vi "Jet_Input.vi"(4 "error in (no error)":errorcluster, 5 "Measured origin x,y":dbl[](array[numeric])=[0.83, 0.79], 6 "Element In":T6, 7 "Outputmode":u16(ring) items=["Get Path", "Make Layout", "Create TRJs"]) -> (0 "error out":errorcluster, 1 "Init Cluster":T8, 2 "TRJs":T5, 3 "Elements out":T7(array[cluster]))   [LabVIEW 2009]
panel:
  out "output cluster":T1
  in  "Tab Control":enum32{"Main", "Expert", "Output"}(tab)=enum."Output"
  out "Tube length":dbl=7.947000000000001
  in  "Ab rate tube":dbl=0.016
  in  "Laser interval tube":dbl=0.01
  in  "Hight to groove(tube center)":dbl=3.0
  in  "Origin to jet outlet (Jet toal)":dbl=10.0
  in  "stop":bool
  in  "Machining geometry (mm)":T2={"a0 radius"=0.35, "a0 depth"=0.5, "b0 radius"=0.1, "b0(depth)"=0.15, "a1 radius"=0.2, "a1 depth"=0.3}
  in  "Length":T3={" l0"=0.5, "l1"=0.35, "l 2"=0.5, "l 3"=0.5}
  out "jet head  length":dbl=1.853
  in  "Gap between  \nl1 and l2":dbl=0.003
  in  "Laser interval jet":dbl=0.008
  in  "Ab rate jet":dbl=0.01
  out "Drawing":picture
  in  "XY Line Arc Trajectory tube":T4={"Velocity (units/s)"=3.0, "Acceleration (unts/s2)"=20.0, "Number of times of execution"=1} {"Acceleration (unts/s2)" format="%.6f"; "Velocity (units/s)" format="%.6f"; "Number of times of execution" format="%.6f"}
  in  "XY Line Arc Trajectory jet":T4={"Velocity (units/s)"=3.0, "Acceleration (unts/s2)"=20.0, "Number of times of execution"=1} {"Acceleration (unts/s2)" format="%.6f"; "Velocity (units/s)" format="%.6f"; "Number of times of execution" format="%.6f"}
  in  "Type":i32=2
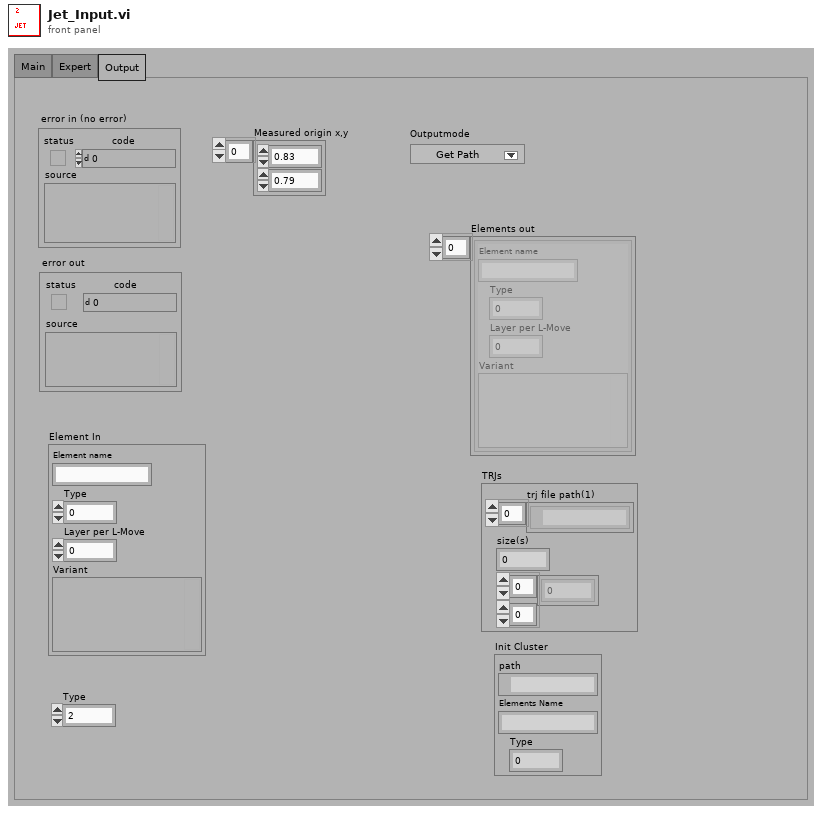
[diagram p1: front panel]
types:
  T1 = cluster{"Hight to groove(tube center)":dbl, "Origin to jet outlet (Jet toal)":dbl, "Laser interval tube":dbl, "Ab rate tube":dbl, "Machining geometry (mm)":cluster{"a0 radius":dbl, "a0 depth":dbl, "b0 radius":dbl, "b0(depth)":dbl, "a1 radius":dbl, "a1 depth":dbl}, "Gap between  \nl1 and l2 ":dbl, "Length":cluster{" l0":dbl, "l1":dbl, "l 2":dbl, "l 3":dbl}, "Laser interval jet":dbl, "Ab rate jet":dbl, "XY Line Arc Trajectory tube":cluster{"Velocity (units/s)":dbl, "Acceleration (unts/s2)":dbl, "Number of times of execution":i32}, "XY Line Arc Trajectory jet":cluster{"Velocity (units/s)":dbl, "Acceleration (unts/s2)":dbl, "Number of times of execution":i32}, "Part #":dbl}
  T2 = cluster{"a0 radius":dbl, "a0 depth":dbl, "b0 radius":dbl, "b0(depth)":dbl, "a1 radius":dbl, "a1 depth":dbl}
  T3 = cluster{" l0":dbl, "l1":dbl, "l 2":dbl, "l 3":dbl}
  T4 = cluster{"Velocity (units/s)":dbl, "Acceleration (unts/s2)":dbl, "Number of times of execution":i32}
  T5 = cluster{"trj file path(1)":path[], "size(s)":i32, dbl[][]}
  T6 = cluster{"Element name":string, "Type":i32, "Layer per L-Move":i32, "Variant":variant}
  T7 = cluster{"Element name":string, "Type":i32, "Layer per L-Move":i32, "Variant":variant}[]
  T8 = cluster{"path":path, "Elements Name":string, "Type":i32}
  T9 = cluster{"path":path, "Button Name":string, "Type":i32}
  T10 = cluster{"Element name":string, "Value":i32, "Layer per L-Move":i32, "Variant":variant}
  T11 = cluster{"Element name":string, "Value":i32, "Layer per L-Move":i32, "Variant":variant}[]
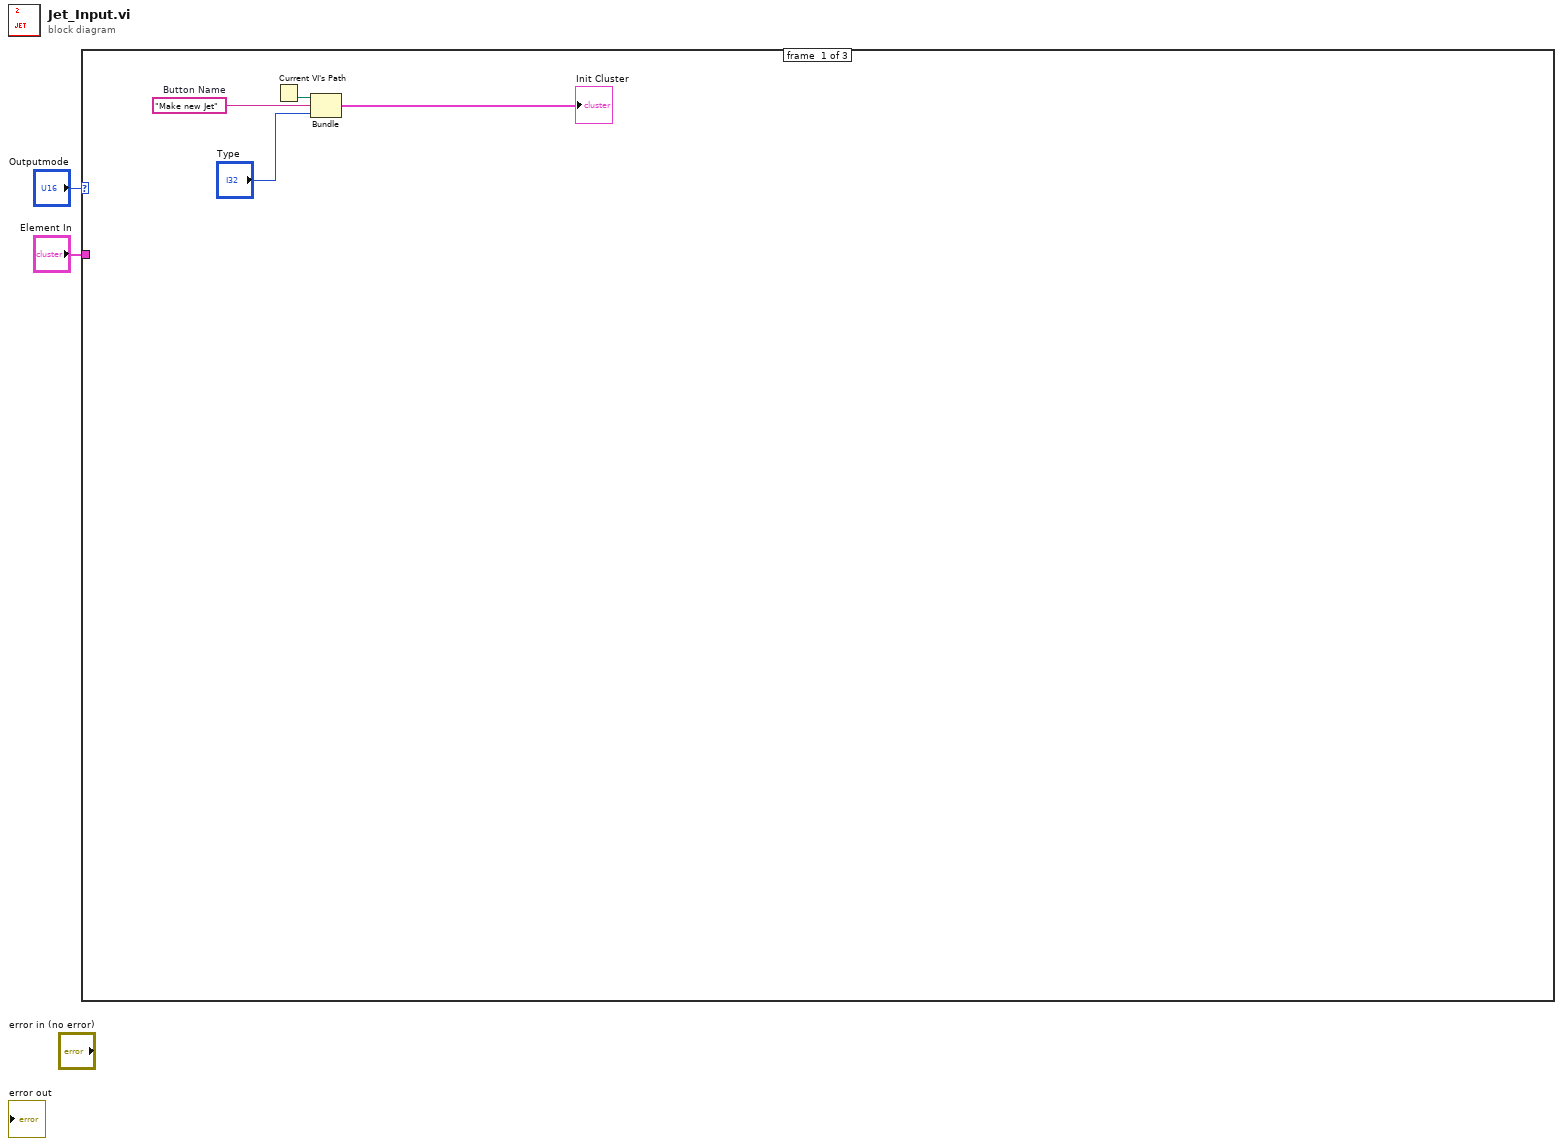
[diagram p0: block diagram]
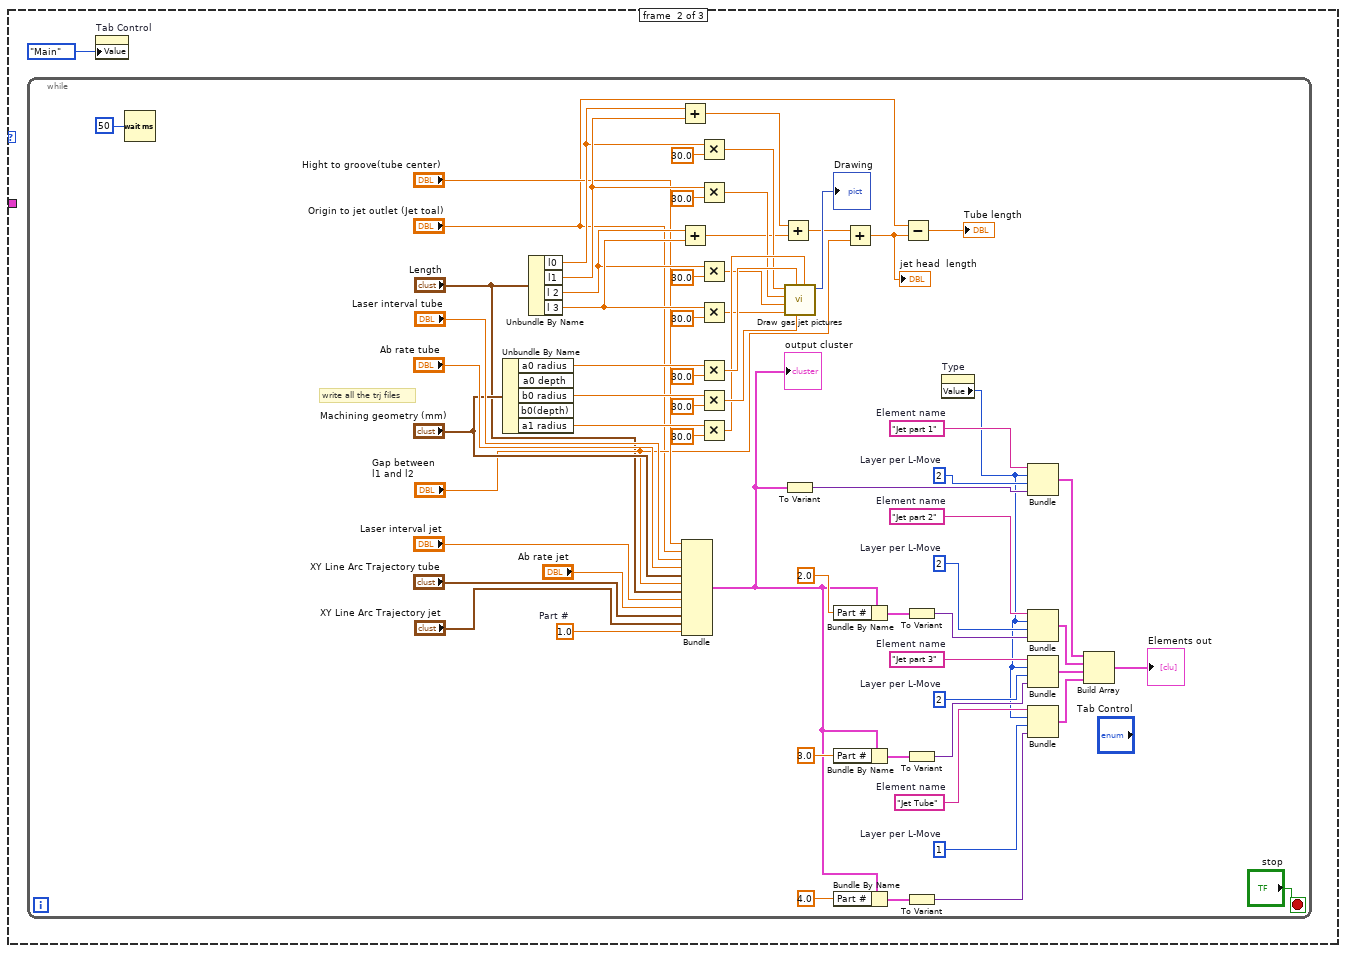
[diagram p2: hidden frame]
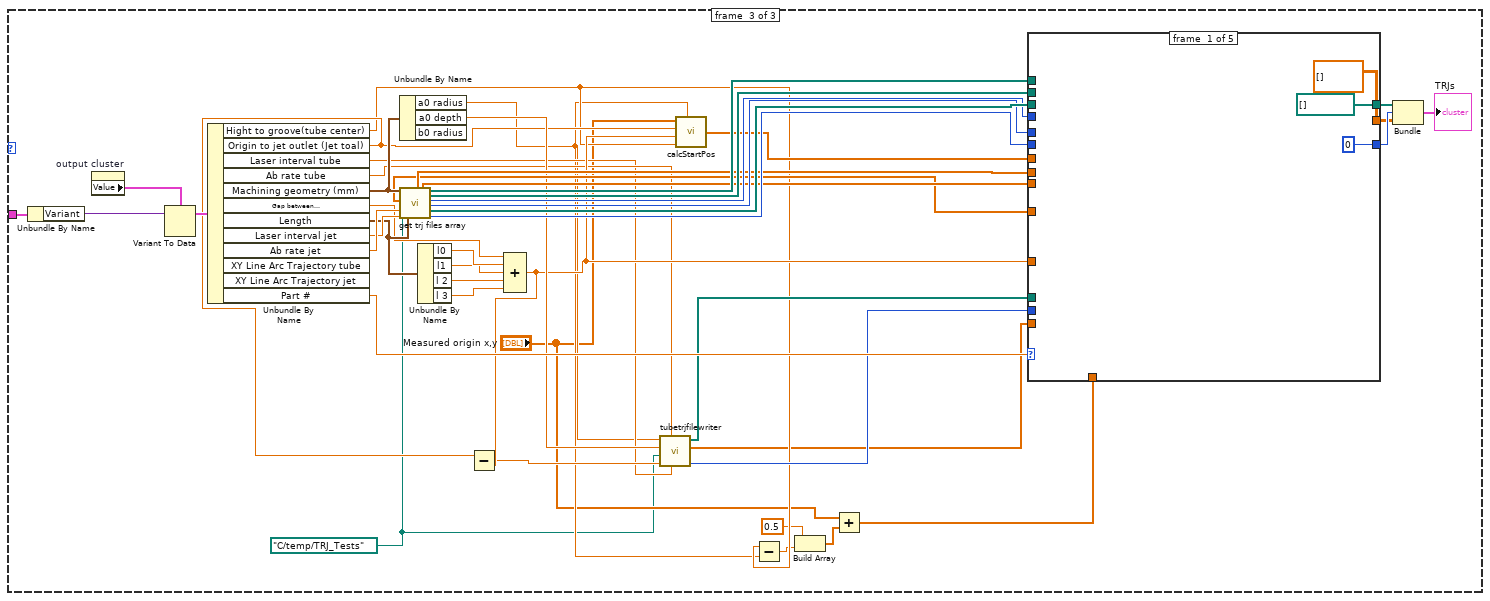
[diagram p3: hidden frame]
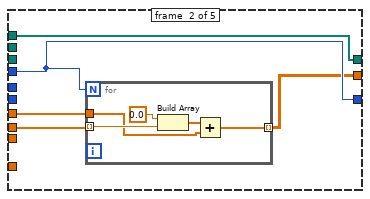
[diagram p4: hidden frame]
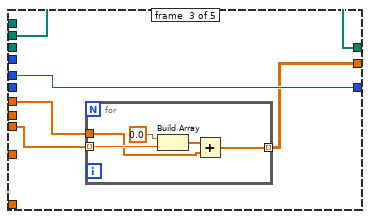
[diagram p5: hidden frame]
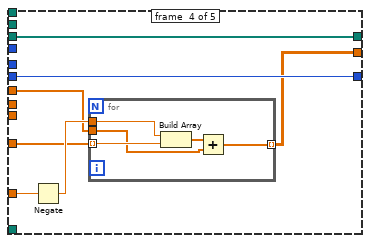
[diagram p6: hidden frame]
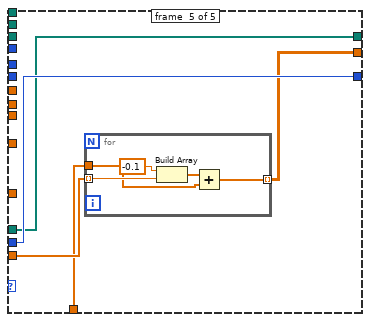
[diagram p7: hidden frame]
diagram:
  n1 = case shown="2" "Outputmode" {
    tunnel: "Element In" -> [_ _ w118]
    frame #0 {
      w6 = "Make new Jet"  # Button Name
      n2 = Current VI's Path() -> (path=w5:path)
      n3 = Bundle("path"=w5, "Button Name"=w6, "Type"="Type") -> (→"Init Cluster":T9)  [unwired: 1 in]
    }
    frame #1 {
      n4 = while {
        stop <- "stop" stop-if-true
        w21 = 1  # Layer per L-Move
        w20 = "Jet Tube"  # Element name
        w22 = 2  # Layer per L-Move
        w23 = "Jet part 3"  # Element name
        w27 = 2  # Layer per L-Move
        w26 = "Jet part 2"  # Element name
        w30 = 1.0  # Part #
        w31 = 2  # Layer per L-Move
        w32 = "Jet part 1"  # Element name
        # "write all the trj files"
        n5 = Wait (ms)(milliseconds to wait=u32 50) -> ()  [unwired: 1 out]
        n6 = Unbundle By Name("Machining geometry (mm)") -> ("a0 radius"=w71:dbl, "b0 radius"=w70:dbl, "a1 radius"=w69:dbl)  [unwired: 2 out]
        n7 = Unbundle By Name("Length") -> ("l0"=w57:dbl, "l1"=w58:dbl, "l 2"=w59:dbl, "l 3"=w60:dbl)
        n8 = Add(x=w57, y=w58) -> (x+y=w47:dbl)
        n9 = Add(x=w59, y=w60) -> (x+y=w48:dbl)
        n10 = Bundle("Hight to groove(tube center)"="Hight to groove(tube center)", "Origin to jet outlet (Jet toal)"="Origin to jet outlet (Jet toal)", "Laser interval tube"="Laser interval tube", "Ab rate tube"="Ab rate tube", "Machining geometry (mm)"="Machining geometry (mm)", "Gap between  \nl1 and l2"="Gap between  \nl1 and l2", "Length"="Length", "Laser interval jet"="Laser interval jet", "Ab rate jet"="Ab rate jet", "XY Line Arc Trajectory tube"="XY Line Arc Trajectory tube", "XY Line Arc Trajectory jet"="XY Line Arc Trajectory jet", "Part #"=w30) -> (w13:T1)  [unwired: 1 in]
        "output cluster" <- w13
        n11 = Multiply(x=w57, y=30.0) -> (x*y=w61:dbl)
        n12 = Multiply(x=w58, y=30.0) -> (x*y=w62:dbl)
        n13 = Multiply(x=w59, y=30.0) -> (x*y=w63:dbl)
        n14 = Multiply(x=w60, y=30.0) -> (x*y=w64:dbl)
        n15 = Multiply(x=w71, y=30.0) -> (x*y=w66:dbl)
        n16 = Multiply(x=w70, y=30.0) -> (x*y=w67:dbl)
        n17 = Multiply(x=w69, y=30.0) -> (x*y=w65:dbl)
        n18 = Add(x=w47, y=w48) -> (x+y=w49:dbl)
        n19 = call "Draw gas jet pictures.vi"("a2"=w65, "b"=w67, "a1"=w66, "l3"=w64, "l2"=w63, "l1"=w62, "l0"=w61) -> ("new picture"=→"Drawing":picture)  [unwired: 4 out]
        n20 = To Variant(anything=w13) -> (Variant=w33:variant)
        n21 = Bundle By Name(cluster=w13, "Part #"=2.0) -> (w17:T1)
        n22 = Bundle By Name(cluster=w13, "Part #"=3.0) -> (w16:T1)
        n23 = Bundle By Name(cluster=w13, "Part #"=4.0) -> (w12:T1)
        n24 = Add(x=w49, y="Gap between  \nl1 and l2") -> (x+y=w35:dbl)
        "jet head  length" <- w35
        n25 = Subtract(x="Origin to jet outlet (Jet toal)", y=w35) -> (x-y=→"Tube length":dbl)
        n26 = To Variant(anything=w17) -> (Variant=w25:variant)
        n27 = To Variant(anything=w16) -> (Variant=w24:variant)
        n28 = To Variant(anything=w12) -> (Variant=w19:variant)
        n29 = property on="Type" class="DigNum (strict)"() -> ("Value"=w8:i32)  [unwired: 2 in, 2 out]
        n30 = Bundle("Element name"=w32, "Value"=w8, "Layer per L-Move"=w31, "Variant"=w33) -> (w29:T10)  [unwired: 1 in]
        n31 = Bundle("Element name"=w26, "Value"=w8, "Layer per L-Move"=w27, "Variant"=w25) -> (w11:T10)  [unwired: 1 in]
        n32 = Bundle("Element name"=w23, "Value"=w8, "Layer per L-Move"=w22, "Variant"=w24) -> (w10:T10)  [unwired: 1 in]
        n33 = Bundle("Element name"=w20, "Value"=w8, "Layer per L-Move"=w21, "Variant"=w19) -> (w9:T10)  [unwired: 1 in]
        n34 = Build Array(w29, w11, w10, w9) -> (→"Elements out":T11)
      }
      n35 = property on="Tab Control" class="TabCtl (strict)"("Value"=enum32{"Main", "Expert", "Output"}."Main" ("Tab Control")) -> ()  [unwired: 2 in, 2 out]
    }
    frame #2 {
      w74 = path "C:/temp/TRJ_Tests" ("file (use dialog)")
      n36 = Unbundle By Name(w118) -> ("Variant"=w117:variant)
      n37 = property on="output cluster" class="Clust (strict)"() -> ("Value"=w116:T1)  [unwired: 2 in, 2 out]
      n38 = Variant To Data(Variant=w117, type=w116) -> (data=w115:T1)  [unwired: 1 in, 1 out]
      n39 = Unbundle By Name(w115) -> ("Hight to groove(tube center)"=w82:dbl, "Origin to jet outlet (Jet toal)"=w89:dbl, "Laser interval tube"=w85:dbl, "Ab rate tube"=w86:dbl, "Machining geometry (mm)"=w98:T2, "Gap between  \nl1 and l2"=w103:dbl, "Length"=w104:T3, "Laser interval jet"=w113:dbl, "Ab rate jet"=w114:dbl, "Part #"=w112:dbl)  [unwired: 2 out]
      n40 = Unbundle By Name(w98) -> ("a0 radius"=w81:dbl, "a0 depth"=w90:dbl)  [unwired: 1 out]
      n41 = call "get trj files array.vi"("Machining geometry (mm)"=w98, "file (use dialog)"=w74, "ab rate"=w114, "interval of  laser path"=w113, "Length(mm)"=w104) -> ("start point  3"=w91:dbl[], "start point 1"=w95:dbl[], "start point  2"=w93:dbl[], "trj file 1"=w111:path[], "trajectory path array 2"=w109:path[], "size1"=w97:i32, "size 2"=w105:i32, "trajectory path array 3"=w108:path[], "size 3"=w106:i32)  [unwired: 6 out]
      n42 = Unbundle By Name(w104) -> ("l0"=w102:dbl, "l1"=w101:dbl, "l 2"=w100:dbl, "l 3"=w99:dbl)
      n43 = Compound Arithmetic op=ADD(w103, w102, w101, w100, w99) -> (w88:dbl)
      n44 = Subtract(x=w89, y=w88) -> (x-y=w87:dbl)
      n45 = call "tubetrjfilewriter.vi"("interval between laser path"=w85, "ablation rate"=w86, "length of capillary"=w87, "file (use dialog)"=w74, "depth"=w90, "radus"=w81) -> ("size(s)"=w83:i32, "start point"=w76:dbl[], "trj file path(1)"=w84:path[])  [unwired: 1 out]
      n46 = call "calcStartPos.vi"("Measured origin x,y"="Measured origin x,y", "Origin to jet outlet (Jet toal)"=w89, "Numeric"=w88, "Hight to groove(tube center)"=w82, "a0 radius"=w81) -> ("Array"=w94:dbl[])
      n47 = Subtract(x=w82, y=w81) -> (x-y=w80:dbl)
      n48 = Build Array(0.5 ("element"), w80) -> (w78:dbl[])
      n49 = Add(x="Measured origin x,y", y=w78) -> (x+y=w75:dbl[])
      n50 = case shown="4" w112 {
        tunnel: w111 -> [_ w126 _ _ _]
        tunnel: [path[] [] ("trj file 1") w126 w136 w148 w157] -> w110
        tunnel: w109 -> [_ _ w136 _ _]
        tunnel: w108 -> [_ _ _ w148 _]
        tunnel: w97 -> [_ w123 _ _ _]
        tunnel: [0 ("size 3") w123 w135 w147 w158] -> w107
        tunnel: w106 -> [_ _ _ w147 _]
        tunnel: w105 -> [_ _ w135 _ _]
        tunnel: w95 -> [_ w125 _ _ _]
        tunnel: w94 -> [_ w124 w133 w144 _]
        tunnel: w93 -> [_ _ w134 _ _]
        tunnel: [dbl[][] [] w122 w132 w142 w154] -> w92
        tunnel: w88 -> [_ _ _ w146 _]
        tunnel: w91 -> [_ _ _ w143 _]
        tunnel: w84 -> [_ _ _ _ w157]
        tunnel: w83 -> [_ _ _ _ w158]
        tunnel: w76 -> [_ _ _ _ w156]
        tunnel: w75 -> [_ _ _ _ w155]
        frame #0 {
        }
        frame #1 {
          n51 = for {
            N: w123 -> [_]
            tunnel: w125 -> [w130] mode=indexing
            tunnel: [w128] -> w122 mode=indexing
            tunnel: w124 -> [w127]
            n52 = Build Array(0.0 ("element"), w130) -> (w129:dbl[])
            n53 = Add(x=w129, y=w127) -> (x+y=w128:dbl[])
          }
        }
        frame #2 {
          n54 = for {
            tunnel: w134 -> [w140] mode=indexing
            tunnel: [w138] -> w132 mode=indexing
            tunnel: w133 -> [w137]
            n55 = Build Array(0.0 ("element"), w140) -> (w139:dbl[])
            n56 = Add(x=w139, y=w137) -> (x+y=w138:dbl[])
          }
        }
        frame #3 {
          n57 = Negate(x=w146) -> (-x=w145:dbl)
          n58 = for {
            tunnel: w143 -> [w153] mode=indexing
            tunnel: [w151] -> w142 mode=indexing
            tunnel: w144 -> [w150]
            tunnel: w145 -> [w149]
            n59 = Build Array(w149, w153) -> (w152:dbl[])
            n60 = Add(x=w152, y=w150) -> (x+y=w151:dbl[])
          }
        }
        frame #4 {
          n61 = for {
            tunnel: w156 -> [w162] mode=indexing
            tunnel: [w160] -> w154 mode=indexing
            tunnel: w155 -> [w159]
            n62 = Build Array(-0.1 ("element"), w162) -> (w161:dbl[])
            n63 = Add(x=w161, y=w159) -> (x+y=w160:dbl[])
          }
        }
      }
      n64 = Bundle("trj file path(1)"=w110, "size(s)"=w107, w92) -> (→"TRJs":T5)  [unwired: 1 in]
    }
  }
